vi "FPGA Calibration.vi"(8 "error in":errorcluster, 11 "FPGA Interface":T1) -> (0 "error out":errorcluster, 3 "FPGA Interface 2":T1)   [LabVIEW 2015]
uses:
  Formula Hybrid 2012 r1/FPGA Typedef.ctl
  <vilib>/rvi/errors/niLvFpgaAdjustHostInterfaceError.vi
  <vilib>/Utility/error.llb/Error Cluster From Error Code.vi
  <vilib>/rvi/interface/nirviReadWriteControl/nirviReadWriteControl.xnode
  FPGA Bitfiles/Latest.lvbitx
  NiFpgaLv.dll
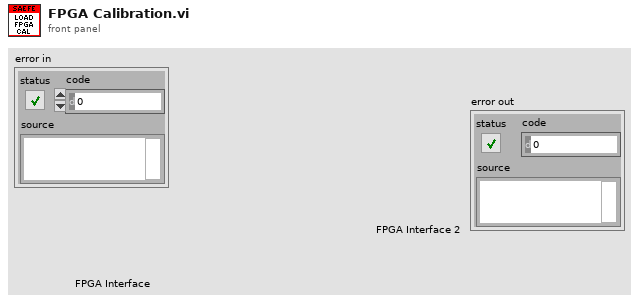
[diagram p1: front panel]
types:
  T1 = typedef "FPGA Typedef.ctl" = refnum<k20>
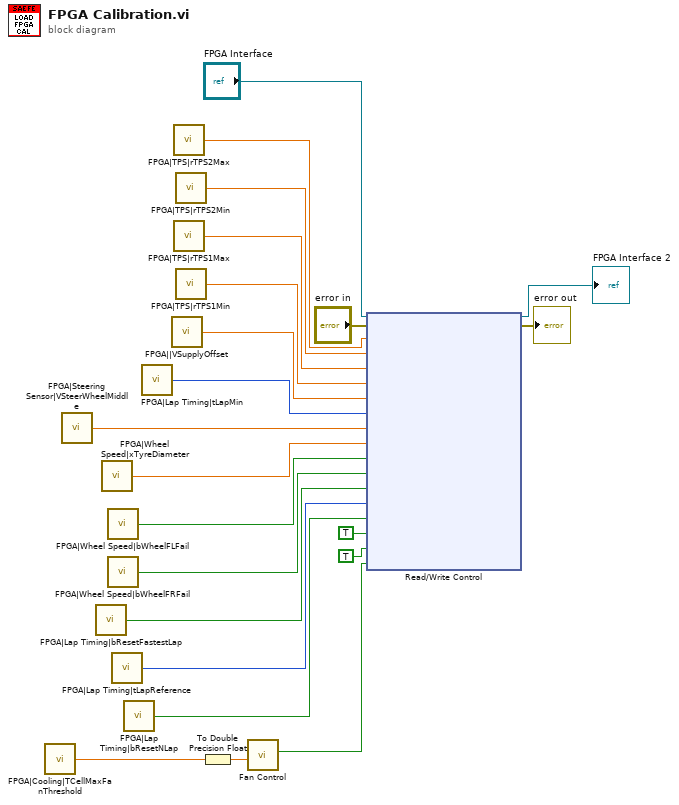
[diagram p0: block diagram]
diagram:
  n1 = call "FPGA|Cooling|TCellMaxFanThreshold"() -> ("Value"=w2:sgl)
  n2 = call "FPGA|Steering Sensor|VSteerWheelMiddle"() -> ("Value"=w14:sgl)
  n3 = call "FPGA|Lap Timing|bResetFastestLap"() -> ("Value"=w10:bool)
  n4 = call "FPGA|Wheel Speed|xTyreDiameter"() -> ("Value"=w13:sgl)
  n5 = call "FPGA|Wheel Speed|bWheelFLFail"() -> ("Value"=w12:bool)
  n6 = call "FPGA|Wheel Speed|bWheelFRFail"() -> ("Value"=w11:bool)
  n7 = call "FPGA|Lap Timing|tLapReference"() -> ("Value"=w9:u32)
  n8 = call "FPGA|Lap Timing|bResetNLap"() -> ("Value"=w8:bool)
  n9 = call "FPGA|Lap Timing|tLapMin"() -> ("Value"=w15:u32)
  n10 = call "FPGA||VSupplyOffset"() -> ("Value"=w16:sgl)
  n11 = call "FPGA|TPS|rTPS2Max"() -> ("Value"=w20:sgl)
  n12 = call "FPGA|TPS|rTPS1Max"() -> ("Value"=w18:sgl)
  n13 = call "FPGA|TPS|rTPS2Min"() -> ("Value"=w19:sgl)
  n14 = call "FPGA|TPS|rTPS1Min"() -> ("Value"=w17:sgl)
  n15 = To Double Precision Float(number=w2) -> (double precision float=w1:dbl)
  n16 = call "Fan Control.vi"("TCellFanStart"=w1) -> ("PWM Out"=w3:bool)  [unwired: 10 in]
  n17 = xnode "Read/Write Control"("FPGA VI Reference In"="FPGA Interface", "error in"="error in", "rTPS2Max"=w20, "rTPS2Min"=w19, "rTPS1Max"=w18, "rTPS1Min"=w17, "VSupplyOffset"=w16, "tLapMin"=w15, "VSteerWheelMiddle"=w14, "Tire Diameter(m)"=w13, "bWheelFLFail"=w12, "bWheelFRFail"=w11, "bResetFastestLap"=w10, "tLapReference"=w9, "bResetNLap"=w8, "bLapBeaconPickupEnable"=TRUE, "bWheelSpeedsEnable"=TRUE, "bAccumulatorFansEnable"=w3) -> ("FPGA VI Reference Out"=→"FPGA Interface 2":T1, "error out"=→"error out":errorcluster)
